vi "AM Proc RES Calculate.vi"(7 "Temp Length":i32[](array[numeric]), 9 "Max Temp Index":i32, 10 "SG at Max Temp":dbl[](array[numeric]), 11 "All Data Cluster":cluster{"Splitted Data":dbl[], dbl[]}[](array[cluster])) -> (3 "Measurement":T2, 6 "Measurement to Show":T1)   [LabVIEW 2020, in "Test Driver.lvlib"]
uses:
  Test Driver.lvlib
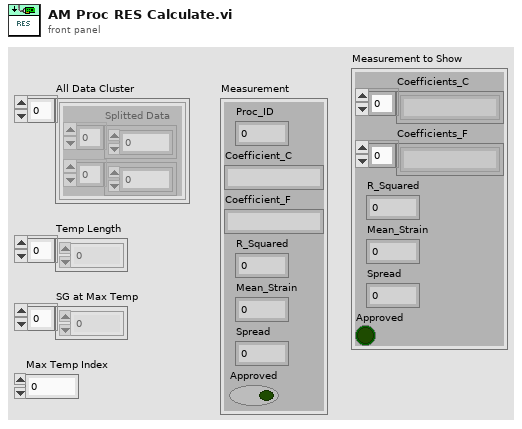
[diagram p1: front panel]
types:
  T1 = cluster{"Coefficients_C":string[], "Coefficients_F":string[], "R_Squared":dbl, "Mean_Strain":dbl, "Spread":dbl, "Approved":bool}
  T2 = cluster{"Proc_ID":i32, "Coefficient_C":string, "Coefficient_F":string, "R_Squared":dbl, "Mean_Strain":dbl, "Spread":dbl, "Approved":bool}
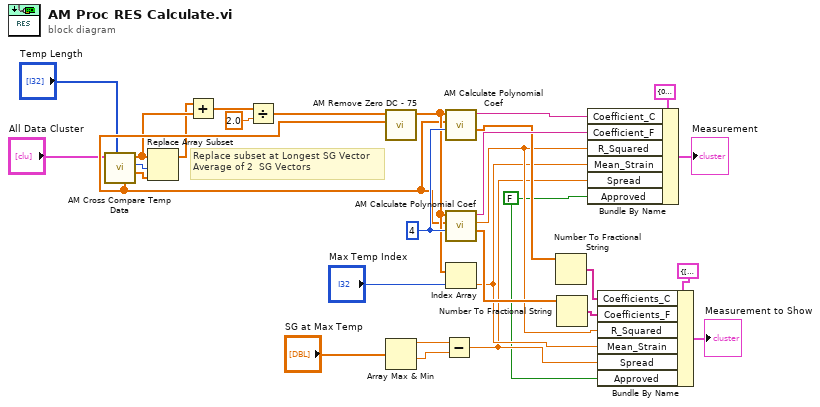
[diagram p0: block diagram]
diagram:
  w2 = FALSE ("Approved")
  w29 = 4 ("polynomial order")
  # "Replace subset at Longest SG Vector\nAverage of 2  SG Vectors"
  n1 = call "AM Cross Compare Temp Data.vi"("Temp Length"="Temp Length", "All Data Cluster"="All Data Cluster") -> ("Small SG Vector"=w18:dbl[], "Cross Index"=w19:i32, "Longest SG Vector"=w20:dbl[], "Longest Temp Vector"=w27:dbl[])  [unwired: 6 in]
  n2 = Replace Array Subset(array=w20, new element=w18, index=w19) -> (w17:dbl[])
  n3 = Add(x=w17, y=w20) -> (x+y=w16:dbl[])
  n4 = Divide(x=w16, y=2.0) -> (x/y=w21:dbl[])
  n5 = call "AM Remove Zero DC - 75.vi"("Longest Temp Vector"=w27, "Average SG"=w21) -> ("normalized SG Data"=w28:dbl[])  [unwired: 9 in]
  n6 = Array Max & Min(array="SG at Max Temp") -> (max value=w23:dbl, min value=w24:dbl)  [unwired: 2 out]
  n7 = Subtract(x=w23, y=w24) -> (x-y=w3:dbl)
  n8 = call "AM Calculate Polynomial Coef.vi"("polynomial order"=w29, "Longest Temp Vector"=w27, "normalized SG Data"=w28) -> ("Polynomial Coefficients"=w9:dbl[], "Polynomial Coefficients Str"=w13:string)  [unwired: 6 in, 1 out]
  n9 = call "AM Calculate Polynomial Coef.vi"("polynomial order"=w29, "Longest Temp Vector"=w27, "normalized SG Data"=w28) -> ("Polynomial Coefficients"=w6:dbl[], "R-square"=w5:dbl, "Polynomial Coefficients Str"=w12:string)  [unwired: 6 in]
  n10 = Index Array(array=w28, index="Max Temp Index") -> (element=w4:dbl)
  n11 = Number To Fractional String(number=w9) -> (F-format string=w8:string[])  [unwired: 3 in]
  n12 = Number To Fractional String(number=w6) -> (F-format string=w7:string[])  [unwired: 3 in]
  n13 = Bundle By Name(cluster=T2 {"Proc_ID"=0, "Coefficient_C"="", "Coefficient_F"="", "R_Squared"=0.0, "Mean_Strain"=0.0, "Spread"=0.0, "Approved"=TRUE} ("Measurement"), "Coefficient_C"=w13, "Coefficient_F"=w12, "R_Squared"=w5, "Mean_Strain"=w4, "Spread"=w3, "Approved"=w2) -> (→"Measurement":T2)
  n14 = Bundle By Name(cluster=T1 {"Coefficients_C"=[], "Coefficients_F"=[], "R_Squared"=0.0, "Mean_Strain"=0.0, "Spread"=0.0, "Approved"=TRUE} ("Procedure Results"), "Coefficients_C"=w8, "Coefficients_F"=w7, "R_Squared"=w5, "Mean_Strain"=w4, "Spread"=w3, "Approved"=w2) -> (→"Measurement to Show":T1)
